vi "CleanUp.vi"(0 "class data in":refnum<class "SceneRoot.lvclass">, 5 "error in":errorcluster) -> (14 "class data out":refnum<class "SceneRoot.lvclass">, 19 "error out":errorcluster)   [LabVIEW 2010, in "RenderBase.lvlib" / "SceneRoot.lvclass"]
doc: "Closes open references."
uses:
  SceneRoot.lvclass
  SceneRoot.lvclass/SceneRoot.ctl
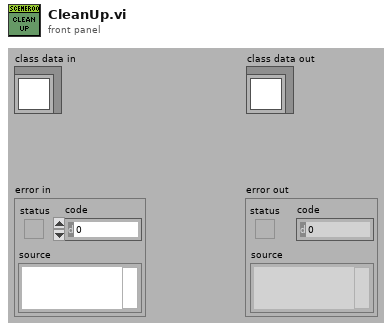
[diagram p1: front panel]
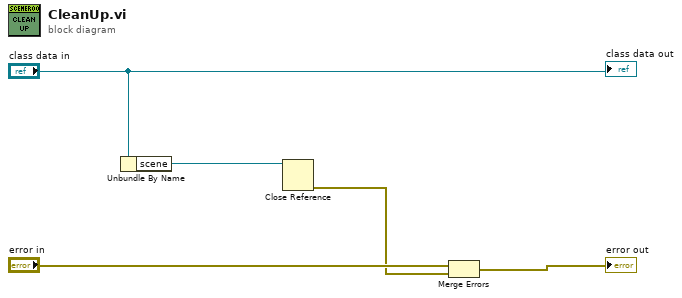
[diagram p0: block diagram]
diagram:
  n1 = Unbundle By Name("class data in") -> ("scene"=w1:refnum<vi>)
  n2 = Close Reference(reference=w1) -> (error out=w3:errorcluster)  [unwired: 1 in]
  n3 = Merge Errors("error in", w3) -> (→"error out":errorcluster)
  "class data out" <- "class data in"
